vi "FTW-JSON-Duplicate.vi"(0 "JSON Object":refnum<data-value>, 11 "error in":errorcluster) -> (4 "JSON Object out":refnum<data-value>, 6 "Duplicated JSON Object":refnum<data-value>, 15 "error out":errorcluster)   [LabVIEW 2015]
uses:
  core/FTW-JSON-Core-Structure.ctl
panel:
  # "Inputs"
  # "Outputs"
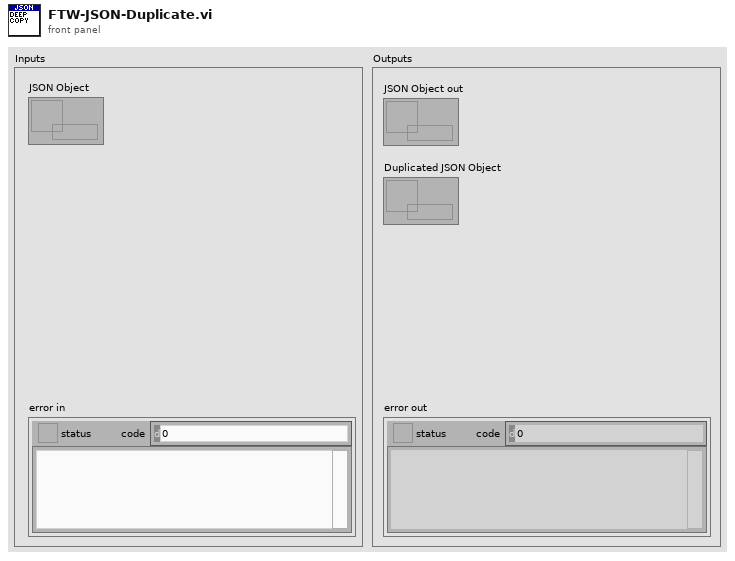
[diagram p1: front panel]
types:
  T1 = typedef "FTW-JSON-Core-Structure.ctl" = cluster{"JSON Object":i64, "Encoding Flags":i64, "Decoding Flags":i64}
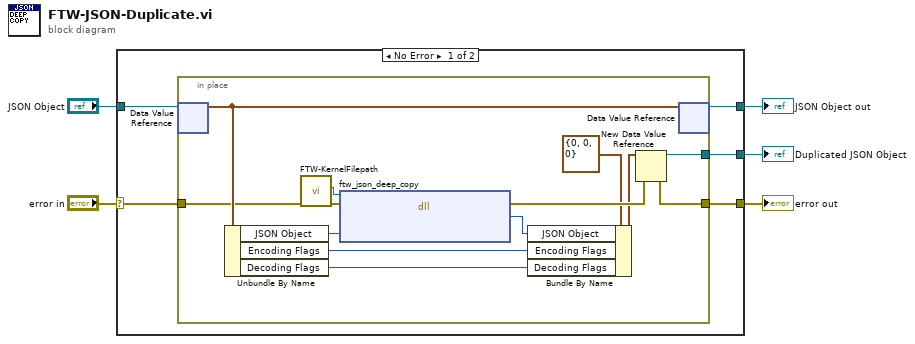
[diagram p0: block diagram]
diagram:
  n1 = case shown="No Error" "error in" {
    selector: "error in" -> [w10 w25]
    tunnel: [w9 w25] -> w5
    tunnel: "JSON Object" -> [w7 w24]
    tunnel: [w6 w24] -> w2
    tunnel: [w8 _] -> w1
    frame No Error {
      n2 = in-place {
        in-place-border: w10 -> [w13]
        in-place-border: [w17] -> w9
        in-place-border: [w19] -> w8
        n3 = in-place-dvr #1(w7) -> (w15:T1)  [unwired: 1 out]
        n4 = Unbundle By Name(w15) -> ("JSON Object"=w23:i64, "Encoding Flags"=w22:i64, "Decoding Flags"=w21:i64)
        n5 = call "FTW-KernelFilepath.vi"("error in"=w13) -> ("error out"=w12:errorcluster, "Library Filepath"=w11:path)  [unwired: 8 in, 1 out]
        n6 = dll-call lib="?" fn="ftw_json_deep_copy"(path in=w11, error in=w12, "Original JSON Object Pointer"=w23) -> (error out=w18:errorcluster, "Duplicate JSON Object Pointer"=w20:i64)  [unwired: 2 in, 1 out]
        n7 = Bundle By Name(cluster=T1 {"JSON Object"=0, "Encoding Flags"=0, "Decoding Flags"=0} ("data value"), "JSON Object"=w20, "Encoding Flags"=w22, "Decoding Flags"=w21) -> (w16:T1)
        n8 = New Data Value Reference(data value=w16, error in=w18) -> (data value reference=w19:refnum<data-value>, error out=w17:errorcluster)
        n9 = in-place-dvr #1(w15) -> (w6:refnum<data-value>)  [unwired: 1 out]
      }
    }
    frame Error {
    }
  }
  "error out" <- w5
  "Duplicated JSON Object" <- w1
  "JSON Object out" <- w2
